vi "Periodic Tasks.vi"() -> ()   [LabVIEW 2011]
doc: "This VI runs in parallel to other tasks. It can contain as many user-defined periodic loops as you need. These can carry out PID or other sorts of timed response."
uses:
  <vilib>/Rock Robotics/SystemInterfaces/Utilities/FPGA_UtilitiesLED State.ctl
  <vilib>/Rock Robotics/SystemInterfaces/Utilities/FPGA_UtilitiesLED Source.ctl
  GLOBALMain.vi
  GLOBALHarvester.vi
  GLOBALShooter.vi
  GLOBALBridge.vi
  GLOBALDriver.vi
  Robot Global Data.vi
panel:
  out "Right Rate":dbl
  out "Right Direction":bool
  out "Right Distance":dbl
  out "Shooter Encoder Distance":dbl
  out "Shooter Direction":bool
  out "Shooter Encoder Rate":dbl
  out "Left Rate":dbl
  out "Gyro Rate":dbl
  out "Gyro Angle":dbl
  out "Left Direction":bool
  out "Left Distance":dbl
  # "Sensor Feedback"
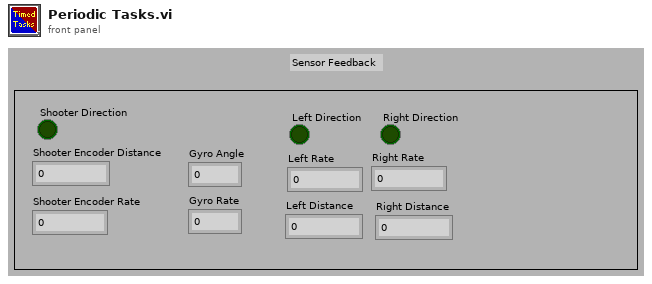
[diagram p1: front panel]
types:
  T1 = typedef "FPGA_UtilitiesLED State.ctl" = enum16{"Off", "On", "Toggle"}
  T2 = typedef "FPGA_UtilitiesLED Source.ctl" = enum16{"User LED", "FPGA LED"}
  T3 = typedef "WPI_AnalogChannelDevRef.ctl" = cluster{"DevStatus":errorcluster, "Analog Module":T4, "Analog Channel":T5}
  T4 = typedef "FPGA_TypedefAnalogModule.ctl" = enum16{"Analog Module 1", "Analog Module 2"}
  T5 = typedef "FPGA_AIChannel.ctl" = enum8{"AI 1", "AI 2", "AI 3", "AI 4", "AI 5", "AI 6", "AI 7", "AI 8", "Invalid"}
  T6 = typedef "WPI_GyroDevRef.ctl" = cluster{"DevStatus":errorcluster, "Analog Module":T4, "Analog Channel":T5, "Offset":dbl, "Gain (VoltsPerDegree/Second)":dbl}
  T7 = typedef "WPI_EncoderDevRef.ctl" = cluster{"DevStatus":errorcluster, "EncoderIndex":T8, "CounterIndex":T9, "DistancePerCount":dbl, "Decoding Type":T10}
  T8 = typedef "FPGA_EncoderIdx.ctl" = enum8{"Enc 0", "Enc 1", "Enc 2", "Enc 3", "Invalid"}
  T9 = typedef "FPGA_CounterCtrSystemIndex.ctl" = enum8{"Ctr 0", "Ctr 1", "Ctr 2", "Ctr 3", "Ctr 4", "Ctr 5", "Ctr 6", "Ctr 7", "Invalid"}
  T10 = typedef "WPI_EncoderType.ctl" = enum16{"1x", "2x", "4x"}
  T11 = typedef "WPI_RelayDevRef.ctl" = cluster{"DevStatus":errorcluster, "Relay Channel":T12, "Digital Module":T13, "Relay Direction":T14}
  T12 = typedef "FPGA_DIORelayChannel.ctl" = enum8{"Relay 1", "Relay 2", "Relay 3", "Relay 4", "Relay 5", "Relay 6", "Relay 7", "Relay 8", "Invalid"}
  T13 = typedef "FPGA_TypedefDigitalModule.ctl" = enum16{"Digital Module 1", "Digital Module 2"}
  T14 = typedef "WPI_RelayDirection.ctl" = enum16{"Both directions", "Forward only", "Reverse only"}
  T15 = typedef "WPI_RelayValue.ctl" = enum16{"Off", "On", "Forward", "Reverse"}
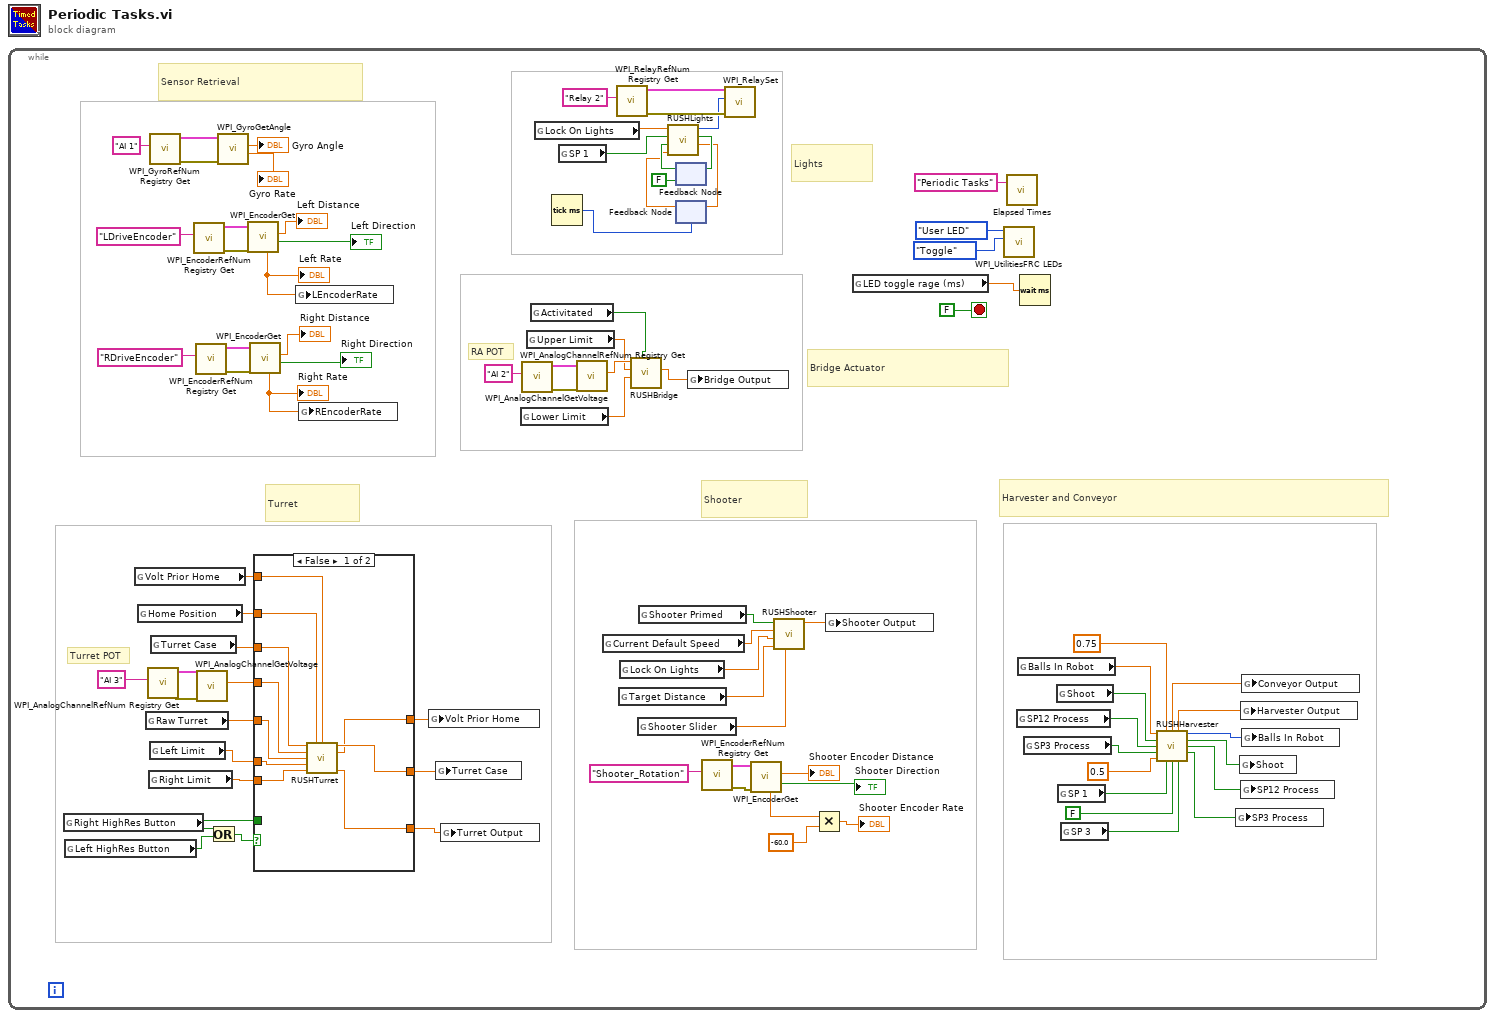
[diagram p0: block diagram]
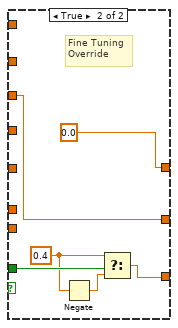
[diagram p2: hidden frame]
diagram:
  n1 = while {
    stop <- FALSE stop-if-true
    # "Lights"
    # "RA POT"
    # "Turret POT"
    # "Harvester and Conveyor"
    # "Shooter"
    # "Sensor Retrieval"
    # "Turret"
    # "Bridge Actuator"
    n2 = global read "GLOBALDriver.vi" "Right HighRes Button"() -> (w45:bool)
    n3 = global read "GLOBALDriver.vi" "Left HighRes Button"() -> (w42:bool)
    n4 = global read "GLOBALShooter.vi" "Volt Prior Home"() -> (w56:dbl)
    n5 = global read "GLOBALShooter.vi" "Home Position"() -> (w55:dbl)
    n6 = global read "GLOBALShooter.vi" "Raw Turret"() -> (w52:dbl)
    n7 = call <vilib>:"WPI_AnalogChannelRefNum Registry Get.vi"("refnum name"="AI 3") -> ("error out"=w48:errorcluster, "AIDeviceRef"=w47:T3)  [unwired: 9 in]
    n8 = global read "GLOBALShooter.vi" "Right Limit"() -> (w53:dbl)
    n9 = call <vilib>:"WPI_GyroRefNum Registry Get.vi"("refnum name"="AI 1") -> ("error out"=w84:errorcluster, "GyroDevRef"=w85:T6)  [unwired: 9 in]
    n10 = global read "GLOBALShooter.vi" "Left Limit"() -> (w54:dbl)
    n11 = global read "GLOBALShooter.vi" "Turret Case"() -> (w50:dbl)
    n12 = call <vilib>:"WPI_EncoderRefNum Registry Get.vi"("refnum name"="LDriveEncoder") -> ("error out"=w79:errorcluster, "EncoderDevRef"=w78:T7)  [unwired: 9 in]
    n13 = call <vilib>:"WPI_EncoderRefNum Registry Get.vi"("refnum name"="RDriveEncoder") -> ("error out"=w73:errorcluster, "EncoderDevRef"=w72:T7)  [unwired: 9 in]
    n14 = call <vilib>:"WPI_AnalogChannelGetVoltage.vi"("error in (no error)"=w48, "AIDeviceRef"=w47) -> ("Voltage"=w49:dbl)  [unwired: 7 in, 2 out]
    n15 = Or(x=w45, y=w42) -> (x .or. y?=w43:bool)
    n16 = call <vilib>:"WPI_GyroGetAngle.vi"("error in (no error)"=w84, "GyroDevRef"=w85) -> ("Angular Rate"=→"Gyro Rate":dbl, "Angle"=→"Gyro Angle":dbl)  [unwired: 6 in, 2 out]
    n17 = call <vilib>:"WPI_EncoderGet.vi"("error in (no error)"=w79, "EncoderDevRef"=w78) -> ("Direction"=→"Left Direction":bool, "Distance"=→"Left Distance":dbl, "Rate"=w75:dbl)  [unwired: 4 in, 3 out]
    "Left Rate" <- w75
    n18 = call <vilib>:"WPI_EncoderGet.vi"("error in (no error)"=w73, "EncoderDevRef"=w72) -> ("Direction"=→"Right Direction":bool, "Distance"=→"Right Distance":dbl, "Rate"=w69:dbl)  [unwired: 4 in, 3 out]
    "Right Rate" <- w69
    n19 = case shown="False" w43 {
      tunnel: [w96 w100] -> w44
      tunnel: w45 -> [_ w103]
      tunnel: w49 -> [w94 _]
      tunnel: w50 -> [w93 w98]
      tunnel: [w97 w98] -> w51
      tunnel: w52 -> [w95 _]
      tunnel: w53 -> [w92 _]
      tunnel: w54 -> [w91 _]
      tunnel: w55 -> [w90 _]
      tunnel: w56 -> [w89 _]
      tunnel: [w88 0.0] -> w57
      frame False {
        n20 = call "RUSHTurret.vi"("Case"=w93, "Home Position"=w90, "Volt Prior Home"=w89, "POT"=w94, "Raw Turret"=w95, "Left Limit"=w91, "Right Limit"=w92) -> ("New Case"=w97:dbl, "Volt prior home"=w88:dbl, "Output"=w96:dbl)  [unwired: 6 in]
      }
      frame True {
        w101 = 0.4 ("t")
        # "Fine Tuning\nOverride"
        n21 = Negate(x=w101) -> (-x=w102:dbl)
        n22 = Select(t=w101, s=w103, f=w102) -> (s? t:f=w100:dbl)
      }
    }
    n23 = global write "Robot Global Data.vi" "LEncoderRate"(w75) -> ()
    n24 = global write "Robot Global Data.vi" "REncoderRate"(w69) -> ()
    n25 = global write "GLOBALShooter.vi" "Volt Prior Home"(w57) -> ()
    n26 = global write "GLOBALShooter.vi" "Turret Case"(w51) -> ()
    n27 = global write "GLOBALShooter.vi" "Turret Output"(w44) -> ()
    n28 = global read "GLOBALBridge.vi" "Lower Limit"() -> (w20:dbl)
    n29 = call <vilib>:"WPI_AnalogChannelRefNum Registry Get.vi"("refnum name"="AI 2") -> ("error out"=w66:errorcluster, "AIDeviceRef"=w67:T3)  [unwired: 9 in]
    n30 = global read "GLOBALBridge.vi" "Upper Limit"() -> (w19:dbl)
    n31 = global read "GLOBALBridge.vi" "Activitated"() -> (w18:bool)
    n32 = global read "GLOBALShooter.vi" "Lock On Lights"() -> (w12:dbl)
    n33 = Tick Count (ms)() -> (millisecond timer value=w7:u32)
    n34 = global read "GLOBALHarvester.vi" "SP 1"() -> (w11:bool)
    n35 = call <vilib>:"WPI_AnalogChannelGetVoltage.vi"("error in (no error)"=w66, "AIDeviceRef"=w67) -> ("Voltage"=w21:dbl)  [unwired: 7 in, 2 out]
    n36 = global read "GLOBALShooter.vi" "Current Default Speed"() -> (w37:dbl)
    n37 = call <vilib>:"WPI_RelayRefNum Registry Get.vi"("refnum name"="Relay 2") -> ("error out"=w14:errorcluster, "RelayDevRef"=w15:T11)  [unwired: 9 in]
    n38 = global read "GLOBALShooter.vi" "Target Distance"() -> (w39:dbl)
    n39 = global read "GLOBALShooter.vi" "Lock On Lights"() -> (w38:dbl)
    n40 = call "RUSHBridge.vi"("Up to Down"=w18, "RA Down Volt"=w20, "RA Up Volt"=w19, "Voltage"=w21) -> ("Ramp Actuator Ouput"=w17:dbl)  [unwired: 7 in]
    n41 = global read "GLOBALDriver.vi" "Shooter Slider"() -> (w40:dbl)
    n42 = global read "GLOBALShooter.vi" "Shooter Primed"() -> (w36:bool)
    n43 = feedback #1(FALSE ("Output")) -> (w9:bool)
    n44 = feedback #2(w7) -> (w6:dbl)
    n45 = call "RUSHLights.vi"("In Time"=w6, "Input"=w9, "SP 1"=w11, "Lock On Ligts"=w12) -> ("Out Time"=w5:dbl, "Output"=w10:bool, "RelayValue"=w13:T15)  [unwired: 5 in]
    n46 = feedback-in #1(w10) -> ()
    n47 = feedback-in #2(w5) -> ()
    n48 = global write "GLOBALBridge.vi" "Bridge Output"(w17) -> ()
    n49 = call <vilib>:"WPI_EncoderRefNum Registry Get.vi"("refnum name"="Shooter_Rotation") -> ("error out"=w60:errorcluster, "EncoderDevRef"=w61:T7)  [unwired: 9 in]
    n50 = call <vilib>:"WPI_RelaySet.vi"("error in (no error)"=w14, "RelayValue"=w13, "RelayDevRef"=w15) -> ()  [unwired: 7 in, 2 out]
    n51 = call <vilib>:"WPI_EncoderGet.vi"("error in (no error)"=w60, "EncoderDevRef"=w61) -> ("Direction"=→"Shooter Direction":bool, "Distance"=→"Shooter Encoder Distance":dbl, "Rate"=w58:dbl)  [unwired: 4 in, 3 out]
    n52 = call "RUSHShooter.vi"("Shooter Dial Delta"=w40, "Target Distance"=w39, "Lock On Lights"=w38, "Current Default Speed"=w37, "Shooter Primed"=w36) -> ("Shooter Output"=w41:dbl)  [unwired: 6 in]
    n53 = Multiply(x=w58, y=-60.0) -> (x*y=→"Shooter Encoder Rate":dbl)
    n54 = global write "GLOBALShooter.vi" "Shooter Output"(w41) -> ()
    n55 = global read "GLOBALMain.vi" "LED toggle rage (ms)"() -> (w2:dbl)
    n56 = call <vilib>:"WPI_UtilitiesFRC LEDs.vi"("State"=FPGA_UtilitiesLED_State."Toggle", "LED Type"=FPGA_UtilitiesLED_Source."User LED") -> ()  [unwired: 1 in, 9 out]
    n57 = call "Elapsed Times.vi"("Call Name"="Periodic Tasks") -> ()  [unwired: 2 in, 1 out]
    n58 = global read "GLOBALHarvester.vi" "SP12 Process"() -> (w31:bool)
    n59 = global read "GLOBALHarvester.vi" "Balls In Robot"() -> (w33:dbl)
    n60 = Wait (ms)(milliseconds to wait=w2) -> ()  [unwired: 1 out]
    n61 = global read "GLOBALHarvester.vi" "SP3 Process"() -> (w30:bool)
    n62 = global read "GLOBALHarvester.vi" "Shoot"() -> (w32:bool)
    n63 = global read "GLOBALHarvester.vi" "SP 1"() -> (w29:bool)
    n64 = global read "GLOBALHarvester.vi" "SP 3"() -> (w28:bool)
    n65 = call "RUSHHarvester.vi"("Balls In Robot"=w33, "Speed of Harvester"=0.75 ("Speed of Conveyor"), "Shoot"=w32, "Ball S12 Process"=w31, "Ball S3 Process"=w30, "Speed of Conveyor"=0.5, "SP 1 Triggered"=w29, "SP 2 Triggered"=FALSE, "SP 3 Triggered"=w28) -> ("Conveyer Output"=w23:dbl, "Harvester Output"=w22:dbl, "Balls In Robot Output"=w24:i32, "Shoot Output"=w25:bool, "Ball S12 Process Output"=w26:bool, "Ball S3 Process Output"=w27:bool)  [unwired: 1 in]
    n66 = global write "GLOBALHarvester.vi" "SP3 Process"(w27) -> ()
    n67 = global write "GLOBALHarvester.vi" "Shoot"(w25) -> ()
    n68 = global write "GLOBALHarvester.vi" "Harvester Output"(w22) -> ()
    n69 = global write "GLOBALHarvester.vi" "SP12 Process"(w26) -> ()
    n70 = global write "GLOBALHarvester.vi" "Conveyor Output"(w23) -> ()
    n71 = global write "GLOBALHarvester.vi" "Balls In Robot"(w24) -> ()
  }
